vi "zmq tcp data latency - data request.vi"() -> ()   [LabVIEW 2019]
uses:
  <vilib>/addons/zeromq/socket_type.ctl
  b0abfede-cf44-4378-af0e-b627b2bde918.vi
  7f3c578c-537b-4032-9878-e5b1ee1716e5.vi
  <vilib>/Utility/High Resolution Relative Seconds.vi
  <vilib>/Utility/error.llb/Clear Errors.vi
  <vilib>/addons/zeromq/zmq_context.lvclass
  <vilib>/addons/zeromq/zmq_socket.lvclass
  <vilib>/addons/zeromq/zeromq.lvlib
panel:
  out "I data":sgl[](graph)
  in  "Data to send":enum16{"SGL", "I16"}(ring)
  out "Size":i32 format="%.3pB"
  out "final time":dbl format="%#_6p"
  in  "F 2":sgl=1000000000.0 format="%#_6p"
  in  "F 1":sgl=1000000.0 format="%#_6p"
  in  "Samples":i32=3072000
  in  "endpoint":string="tcp://127.0.0.1:5555"
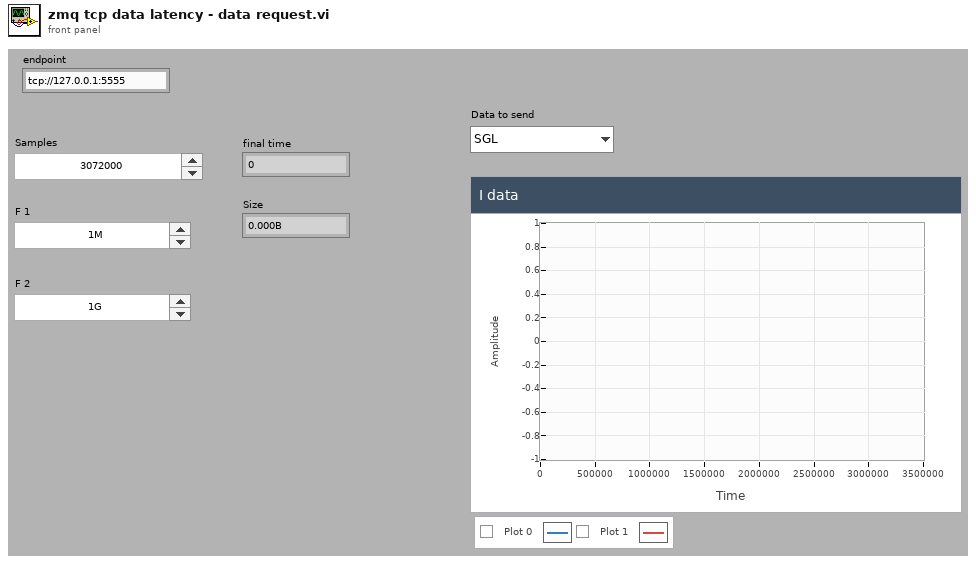
[diagram p1: front panel]
types:
  T1 = typedef "zeromq.lvlib/socket_type.ctl" = enum8{"ZMQ_PAIR", "ZMQ_PUB", "ZMQ_SUB", "ZMQ_REQ", "ZMQ_REP", "ZMQ_DEALER", "ZMQ_ROUTER", "ZMQ_PULL", "ZMQ_PUSH", "ZMQ_XPUB", "ZMQ_XSUB"}
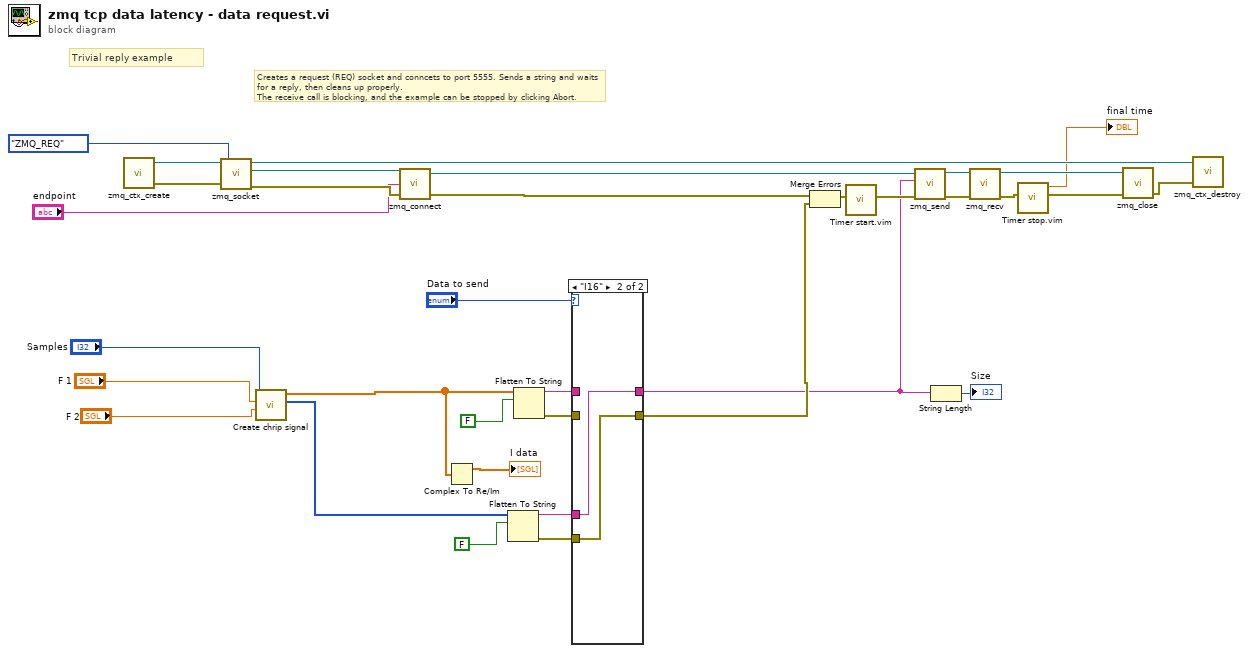
[diagram p0: block diagram]
diagram:
  # "Creates a request (REQ) socket and conncets to port 5555. Sends a string and waits for a reply, then cleans up properly.\nThe receive call is blocking, and the example can be stopped by clicking Abort."
  # "Trivial reply example"
  n1 = call <vilib>:"zmq_ctx_create.vi"() -> ("error out"=w26:errorcluster, "context out"=w34:refnum<class "zmq_context.lvclass">)  [unwired: 4 in]
  n2 = call <vilib>:"zmq_socket.vi"("error in"=w26, "socket type"=socket_type."ZMQ_REQ", "context in"=w34) -> ("error out"=w33:errorcluster, "socket out"=w32:refnum<class "zmq_socket.lvclass">, "context out"=w27:refnum<class "zmq_context.lvclass">)  [unwired: 2 in]
  n3 = call "Create chrip signal.vi"("F 2"="F 2", "F 1"="F 1", "Samples"="Samples") -> ("I16"=w5:i16[], "SGL"=w4:csg[])  [unwired: 7 in]
  n4 = call <vilib>:"zmq_connect.vi"("error in"=w33, "endpoint"="endpoint", "socket in"=w32) -> ("error out"=w22:errorcluster, "socket out"=w31:refnum<class "zmq_socket.lvclass">)  [unwired: 1 in]
  n5 = Complex To Re/Im(x + iy=w4) -> (x=→"I data":sgl[])  [unwired: 1 out]
  n6 = Flatten To String(anything=w5, prepend array or string size? (T)=FALSE) -> (data string=w6:string, error out=w7:errorcluster)  [unwired: 2 in, 1 out]
  n7 = Flatten To String(anything=w4, prepend array or string size? (T)=FALSE) -> (data string=w11:string, error out=w9:errorcluster)  [unwired: 2 in, 1 out]
  n8 = case shown="\"I16\"" "Data to send" {
    tunnel: [w36 w38] -> w8
    tunnel: w11 -> [w36 _]
    tunnel: [w35 w37] -> w10
    tunnel: w9 -> [w35 _]
    tunnel: w6 -> [_ w38]
    tunnel: w7 -> [_ w37]
    frame "SGL", Default {
    }
    frame "I16" {
    }
  }
  n9 = Merge Errors(w22, w10) -> (w18:errorcluster)
  n10 = call "Timer start.vim"("dataflow in"=w18) -> ("dataflow out"=w21:errorcluster)  [unwired: 10 in]
  n11 = call <vilib>:"zmq_send.vi"("error in"=w21, "data"=w8, "socket in"=w31) -> ("error out"=w25:errorcluster, "socket out"=w30:refnum<class "zmq_socket.lvclass">)  [unwired: 4 in]
  n12 = String Length(string=w8) -> (length=→"Size":i32)
  n13 = call <vilib>:"zmq_recv.vi"("error in"=w25, "socket in"=w30) -> ("error out"=w17:errorcluster, "socket out"=w29:refnum<class "zmq_socket.lvclass">)  [unwired: 3 in, 3 out]
  n14 = call "Timer stop.vim"("dataflow in"=w17) -> ("dataflow out"=w15:errorcluster, "final time"=→"final time":dbl)  [unwired: 9 in]
  n15 = call <vilib>:"zmq_close.vi"("error in"=w15, "socket"=w29) -> ("error out"=w28:errorcluster)  [unwired: 3 in]
  n16 = call <vilib>:"zmq_ctx_destroy.vi"("error in"=w28, "context in"=w27) -> ()  [unwired: 3 in, 1 out]
